vi "fgv_XYStage_Move.vi"(10 "Status":enum16{"Initialize", "Write", "Read"}(ring), 11 "XY Stage Move":T1={"Move"=enum."y_line", "max X displacement"=20.0, "max Y displacement"=20.0, "max speed (um/sec)"=500.0, "Move Stage"=FALSE}) -> (3 "XY Stage Move":T1={"Move"=enum."y_line", "max X displacement"=20.0, "max Y displacement"=20.0, "max speed (um/sec)"=500.0, "Move Stage"=FALSE})   [LabVIEW 2020]
uses:
  Typedefs/XY Stage_Move.ctl
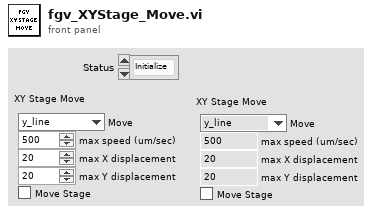
[diagram p1: front panel]
types:
  T1 = typedef "XY Stage_Move.ctl" = cluster{"Move":enum16{"x-line", "y_line", "x-y-line", "random-xy"}, "max X displacement":sgl, "max Y displacement":sgl, "max speed (um/sec)":sgl, "Move Stage":bool}
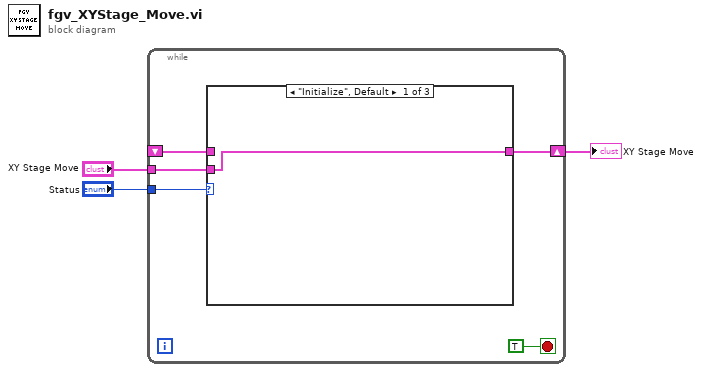
[diagram p0: block diagram]
diagram:
  n1 = while {
    tunnel: "Status" -> [w7]
    shift-right: [w6] -> w1
    shift-left: _ -> [w5]
    tunnel: "XY Stage Move" -> [w4]
    stop <- TRUE stop-if-true
    n2 = case shown="\"Initialize\", Default" w7 {
      tunnel: [w9 w10 w11] -> w6
      tunnel: w5 -> [_ _ w11]
      tunnel: w4 -> [w9 w10 _]
      frame "Initialize", Default {
      }
      frame "Write" {
      }
      frame "Read" {
      }
    }
  }
  "XY Stage Move" <- w1
